vi "Position Attributes.vi"(10 "Speed":i32=10 min=10 max=300 step=1, 11 "Position":dbl min=0.0 max=280.0 step=1.0) -> (2 "params":string, 3 "array":string[](array[string]))   [LabVIEW 2021, in "STAV lib.lvlib"]
uses:
  STAV lib.lvlib
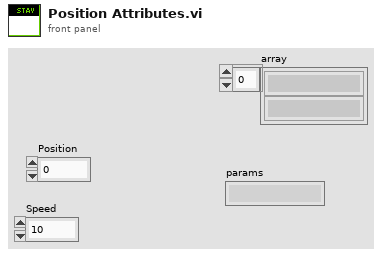
[diagram p1: front panel]
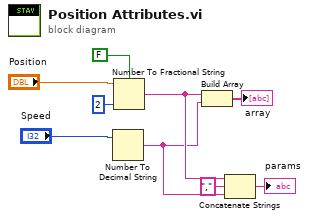
[diagram p0: block diagram]
diagram:
  n1 = Number To Decimal String(number="Speed") -> (decimal integer string=w4:string)  [unwired: 1 in]
  n2 = Number To Fractional String(use system decimal point (T)=FALSE, number="Position", precision (6)=i16 2) -> (F-format string=w5:string)  [unwired: 1 in]
  n3 = Build Array(w5, w4) -> (→"array":string[])
  n4 = Concatenate Strings(w5, "," ("string"), w4) -> (→"params":string)
